vi "Status Msg Joiner v2.vi"(1 "ADD?":bool=TRUE, 2 "Mode":enum16{"Initialize", "Write"}(ring)=enum."Write", 3 "Status Messages":string, 4 "Status Out Ref":refnum<vi>) -> ()   [LabVIEW 2018]
panel:
  out "error out":errorcluster
  out "Status Out":string
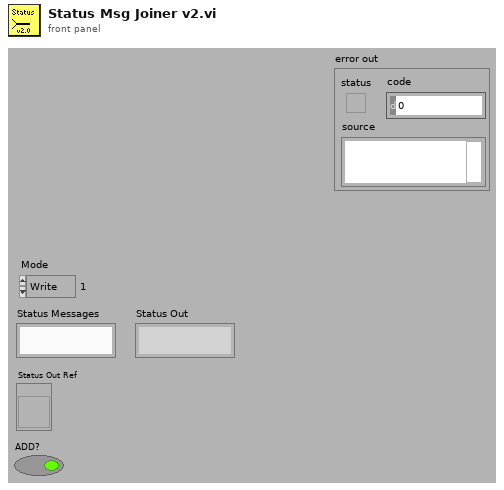
[diagram p1: front panel]
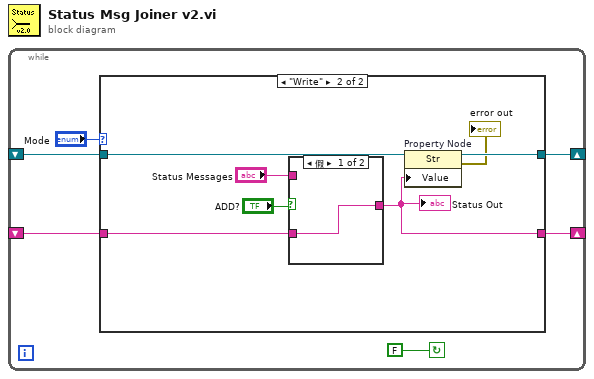
[diagram p0: block diagram]
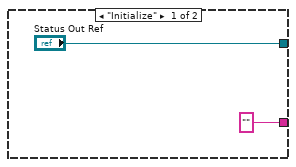
[diagram p2: hidden frame]
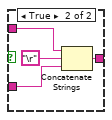
[diagram p3: hidden frame]
diagram:
  n1 = while {
    shift-right: [w4] -> _
    shift-left: _ -> [w3]
    shift-right: [w1] -> _
    shift-left: _ -> [w2]
    stop <- FALSE continue-if-true
    n2 = case shown="\"Write\"" "Mode" {
      tunnel: ["" w13] -> w4
      tunnel: w3 -> [_ w14]
      tunnel: w2 -> [_ w12]
      tunnel: ["Status Out Ref" w11] -> w1
      frame "Initialize" {
      }
      frame "Write" {
        n3 = case shown="假" "ADD?" {
          tunnel: "Status Messages" -> [_ w19]
          tunnel: w14 -> [w16 w18]
          tunnel: [w16 w17] -> w13
          frame False {
          }
          frame True {
            n4 = Concatenate Strings(w19, "\r", w18) -> (w17:string)
          }
        }
        "Status Out" <- w13
        n5 = property on="Property Node" class="Str"(reference=w12, "Value"=w13) -> (reference out=w11:refnum<vi>, error out=→"error out":errorcluster)  [unwired: 1 in]
      }
    }
  }
